vi "Clear Display.vi"(6 "chip select (1st chip)":enum16{"1st chip", "2nd chip"}(ring), 8 "error in (no error)":errorcluster, 11 "LCD in":u32) -> (0 "error out":errorcluster, 3 "LCD out":u32)   [LabVIEW 2015, in "HD44780 FPGA.lvlib"]
doc: "Sets the display data RAM (DDRAM) address 0 into the address counter and returns the display to the original status. This VI also sets the entry mode to increment but keeps the shift setting unchanged."
uses:
  <vilib>/EmbeddedDisplay/Hitachi HD44780/FPGA/HD44780 FPGA.lvlib
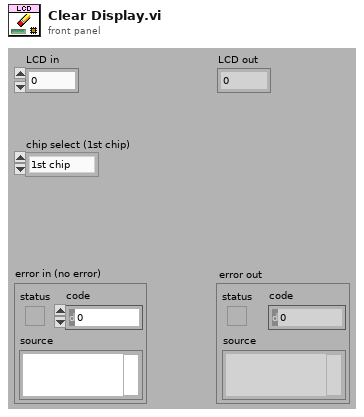
[diagram p1: front panel]
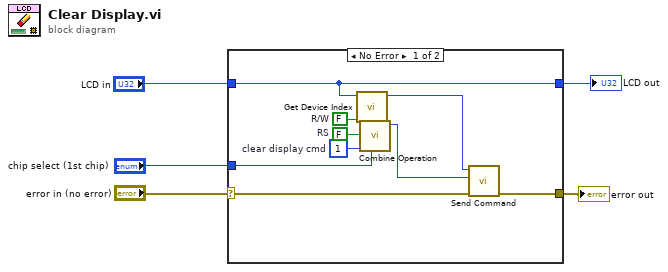
[diagram p0: block diagram]
diagram:
  n1 = case shown="No Error" "error in (no error)" {
    selector: "error in (no error)" -> [w10 w16]
    tunnel: [w9 w16] -> w4
    tunnel: "chip select (1st chip)" -> [w11 _]
    tunnel: "LCD in" -> [w6 w15]
    tunnel: [w6 w15] -> w1
    frame No Error {
      w12 = FALSE  # R/W
      w13 = u8 1  # clear display cmd
      w14 = FALSE  # RS
      n2 = call <vilib>:"Get Device Index.vi"("LCD in"=w6) -> ("device index"=w7:i8)  [unwired: 10 in]
      n3 = call <vilib>:"Combine Operation.vi"("chip select  (1st chip)"=w11, "cmd/data (0)"=w13, "RS"=w14, "R/W"=w12) -> ("output"=w8:u32)  [unwired: 7 in]
      n4 = call <vilib>:"Send Command.vi"("error in (no error)"=w10, "operation"=w8, "device index"=w7) -> ("error out"=w9:errorcluster)  [unwired: 6 in, 2 out]
    }
    frame Error {
    }
  }
  "error out" <- w4
  "LCD out" <- w1
